vi "Configure Probe (Auxiliary).vi"(6 "Auxiliary Operation (0: Setup)":i32(ring) items=["Setup", "Auto Zero", "Degauss"], 7 "Auxiliary Input Mode (1: Pass)":i32(ring)=1 items=["Bypass", "Pass"], 8 "error in (no error)":errorcluster, 9 "Auxiliary Gain (0.1)":dbl=0.1, 10 "Auxiliary Forced Range (0)":dbl, 11 "VISA resource name":refnum<visa-resource-name>) -> (0 "error out":errorcluster, 3 "VISA resource name out":refnum<visa-resource-name>)   [LabVIEW 2017, in "Scope.lvlib" / "Tektronix DPO MSO 2000 4000 Series.lvlib"]
doc: "Configures settings of a probe attached to the auxiliary input for an oscilloscope.\n\n<B>Notes:</B>\nThis VI is available for MSO/DPO4000B series models and 2-channel MDO3000 models only."
uses:
  Tektronix DPO MSO 2000 4000 Series.lvlib
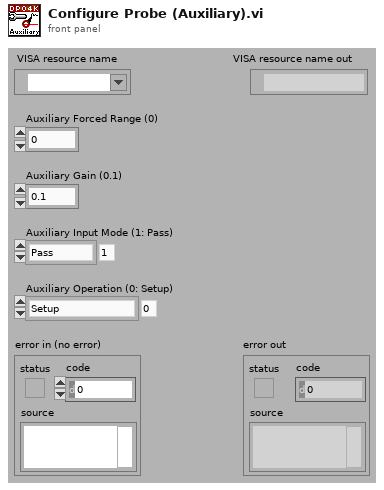
[diagram p1: front panel]
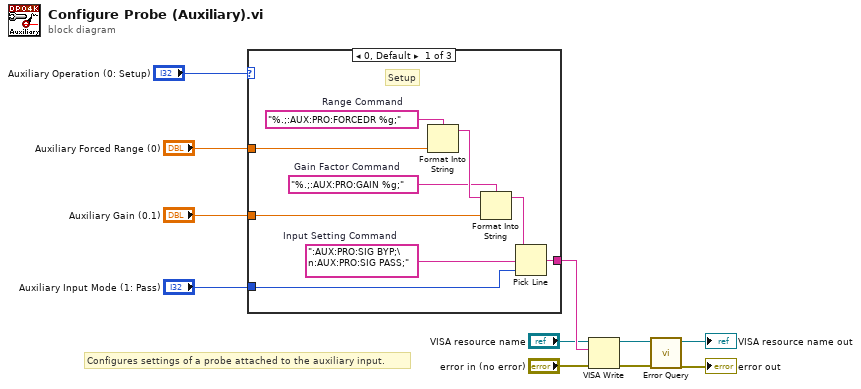
[diagram p0: block diagram]
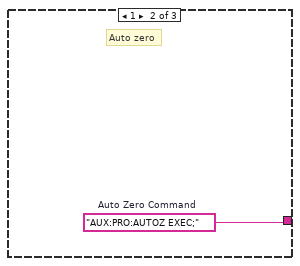
[diagram p2: hidden frame]
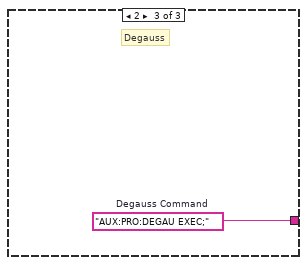
[diagram p3: hidden frame]
diagram:
  # "Configures settings of a probe attached to the auxiliary input."
  n1 = case shown="0, Default" "Auxiliary Operation (0: Setup)" {
    tunnel: "Auxiliary Forced Range (0)" -> [w20 _ _]
    tunnel: "Auxiliary Gain (0.1)" -> [w18 _ _]
    tunnel: "Auxiliary Input Mode (1: Pass)" -> [w17 _ _]
    tunnel: [w15 w21 w22] -> w8
    frame 0, Default {
      w12 = "%.;:AUX:PRO:FORCEDR %g;"  # Range Command
      w13 = "%.;:AUX:PRO:GAIN %g;"  # Gain Factor Command
      w14 = ":AUX:PRO:SIG BYP;\n:AUX:PRO:SIG PASS;"  # Input Setting Command
      # "Setup"
      n2 = Format Into String(format string=w12, w20) -> (resulting string=w19:string)  [unwired: 2 in, 1 out]
      n3 = Format Into String(format string=w13, initial string=w19, w18) -> (resulting string=w16:string)  [unwired: 1 in, 1 out]
      n4 = Pick Line(string ("")=w16, multi-line string=w14, line index=w17) -> (output string=w15:string)
    }
    frame 1 {
      w21 = "AUX:PRO:AUTOZ EXEC;"  # Auto Zero Command
      # "Auto zero"
    }
    frame 2 {
      w22 = "AUX:PRO:DEGAU EXEC;"  # Degauss Command
      # "Degauss"
    }
  }
  n5 = VISA Write(VISA resource name="VISA resource name", write buffer=w8, error in (no error)="error in (no error)") -> (VISA resource name out=w5:refnum<visa-resource-name>, error out=w4:errorcluster)  [unwired: 1 out]
  n6 = call "Error Query.vi"("error in (no error)"=w4, "VISA resource name"=w5) -> ("error out"=→"error out":errorcluster, "VISA resource name out"=→"VISA resource name out":refnum<visa-resource-name>)  [unwired: 6 in, 2 out]
